vi "Move to point.vi"(11 "Point":T1) -> ()   [LabVIEW 2011]
uses:
  point.ctl
  <vilib>/addons/control/pid/pid.llb/PID (DBL).vi
  <vilib>/addons/control/pid/NI_PID_pid.lvlib
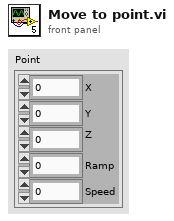
[diagram p1: front panel]
types:
  T1 = typedef "point.ctl" = cluster{"X":dbl, "Y":dbl, "Z":dbl, "Ramp":dbl, "Speed":dbl}
  T2 = typedef "WPI_EncoderDevRef.ctl" = cluster{"DevStatus":errorcluster, "EncoderIndex":T3, "CounterIndex":T4, "DistancePerCount":dbl, "Decoding Type":T5}
  T3 = typedef "FPGA_EncoderIdx.ctl" = enum8{"Enc 0", "Enc 1", "Enc 2", "Enc 3", "Invalid"}
  T4 = typedef "FPGA_CounterCtrSystemIndex.ctl" = enum8{"Ctr 0", "Ctr 1", "Ctr 2", "Ctr 3", "Ctr 4", "Ctr 5", "Ctr 6", "Ctr 7", "Invalid"}
  T5 = typedef "WPI_EncoderType.ctl" = enum16{"1x", "2x", "4x"}
  T6 = typedef "WPI_MotorControlDeviceRef.ctl" = cluster{"DeviceStatus":errorcluster, "Type":enum16{"PWM", "CAN"}, "PWM":cluster{"Digital Module":T7, "PWM Channel":T8, "DeadBand":T9}, "CAN":cluster{"Device Number":u8, "Control Mode":T10, "Semaphore":T11, "Max Vout":dbl}, "Invert":bool, "TransformRef":T12, "InvTransformRef":T12}
  T7 = typedef "FPGA_TypedefDigitalModule.ctl" = enum16{"Digital Module 1", "Digital Module 2"}
  T8 = typedef "FPGA_DIOPWMChannel.ctl" = enum8{"PWM 1", "PWM 2", "PWM 3", "PWM 4", "PWM 5", "PWM 6", "PWM 7", "PWM 8", "PWM 9", "PWM 10", "Invalid"}
  T9 = typedef "WPI_PWMDeadband.ctl" = cluster{"Name":string, "maxPositivePwm":i32, "minPositivePwm":i32, "centerPwm":i32, "maxNegativePwm":i32, "minNegativePwm":i32, "angularRange":u16}
  T10 = typedef "WPI_CANJaguar_ControlMode.ctl" = enum8{"Percent VBus", "Current", "Speed", "Position", "Voltage"}
  T11 = typedef "Semaphore RefNum" = refnum<k1>
  T12 = typedef "WPI_PWMTransform_ConPane.ctl" = refnum<vi>
  T13 = cluster{"proportional gain (Kc)":dbl, "integral time (Ti, min)":dbl, "derivative time (Td, min)":dbl}
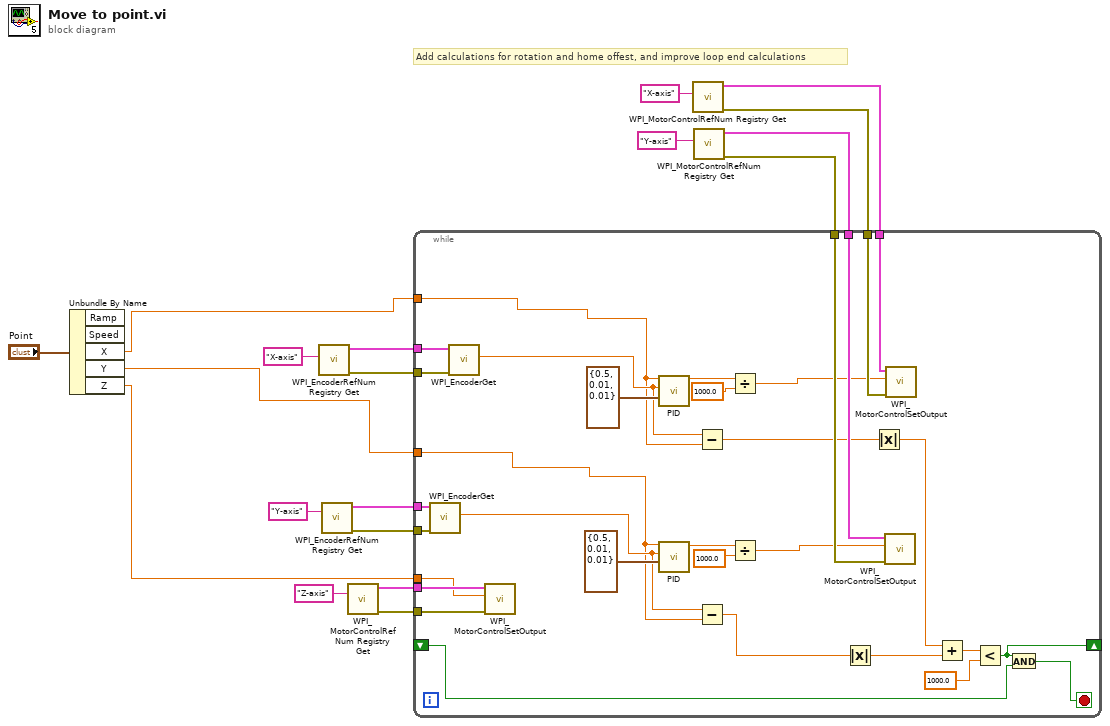
[diagram p0: block diagram]
diagram:
  # "Add calculations for rotation and home offest, and improve loop end calculations"
  n1 = Unbundle By Name("Point") -> ("X"=w1:dbl, "Y"=w2:dbl, "Z"=w3:dbl)  [unwired: 2 out]
  n2 = call <vilib>:"WPI_EncoderRefNum Registry Get.vi"("refnum name"="X-axis") -> ("error out"=w16:errorcluster, "EncoderDevRef"=w15:T2)  [unwired: 9 in]
  n3 = call <vilib>:"WPI_EncoderRefNum Registry Get.vi"("refnum name"="Y-axis") -> ("error out"=w13:errorcluster, "EncoderDevRef"=w14:T2)  [unwired: 9 in]
  n4 = call <vilib>:"WPI_MotorControlRefNum Registry Get.vi"("refnum name"="Z-axis") -> ("error out"=w5:errorcluster, "MotorControlDevRef"=w6:T6)  [unwired: 9 in]
  n5 = call <vilib>:"WPI_MotorControlRefNum Registry Get.vi"("refnum name"="X-axis") -> ("error out"=w10:errorcluster, "MotorControlDevRef"=w11:T6)  [unwired: 9 in]
  n6 = call <vilib>:"WPI_MotorControlRefNum Registry Get.vi"("refnum name"="Y-axis") -> ("error out"=w7:errorcluster, "MotorControlDevRef"=w8:T6)  [unwired: 9 in]
  n7 = while {
    tunnel: w1 -> [w22]
    tunnel: w16 -> [w49]
    tunnel: w15 -> [w48]
    tunnel: w2 -> [w23]
    tunnel: w14 -> [w45]
    tunnel: w13 -> [w44]
    shift-right: [w38] -> _
    shift-left: _ -> [w37]
    tunnel: w11 -> [w36]
    tunnel: w10 -> [w25]
    tunnel: w8 -> [w35]
    tunnel: w7 -> [w34]
    tunnel: w6 -> [w33]
    tunnel: w5 -> [w32]
    tunnel: w3 -> [w24]
    stop <- w26 stop-if-true
    n8 = call <vilib>:"WPI_EncoderGet.vi"("error in (no error)"=w44, "EncoderDevRef"=w45) -> ("Distance"=w27:dbl)  [unwired: 4 in, 5 out]
    n9 = call <vilib>:"WPI_EncoderGet.vi"("error in (no error)"=w49, "EncoderDevRef"=w48) -> ("Distance"=w31:dbl)  [unwired: 4 in, 5 out]
    n10 = call <vilib>:"WPI_MotorControlSetOutput.vi"("error in (no error)"=w32, "Output"=w24, "MotorControlDevRef"=w33) -> ()  [unwired: 7 in, 2 out]
    n11 = call-poly <vilib>:"PID.vi"("PID gains"=T13 {"proportional gain (Kc)"=0.5, "integral time (Ti, min)"=0.01, "derivative time (Td, min)"=0.01}, "process variable"=w31, "setpoint"=w22) -> ("output"=w42:dbl)  [unwired: 7 in, 1 out]
    n12 = call-poly <vilib>:"PID.vi"("PID gains"=T13 {"proportional gain (Kc)"=0.5, "integral time (Ti, min)"=0.01, "derivative time (Td, min)"=0.01}, "process variable"=w27, "setpoint"=w23) -> ("output"=w43:dbl)  [unwired: 7 in, 1 out]
    n13 = Subtract(x=w31, y=w22) -> (x-y=w29:dbl)
    n14 = Subtract(x=w27, y=w23) -> (x-y=w41:dbl)
    n15 = Divide(x=w42, y=1000.0) -> (x/y=w21:dbl)
    n16 = Divide(x=w43, y=1000.0) -> (x/y=w20:dbl)
    n17 = Absolute Value(x=w41) -> (abs(x)=w30:dbl)
    n18 = Absolute Value(x=w29) -> (abs(x)=w28:dbl)
    n19 = call <vilib>:"WPI_MotorControlSetOutput.vi"("error in (no error)"=w34, "Output"=w20, "MotorControlDevRef"=w35) -> ()  [unwired: 7 in, 2 out]
    n20 = call <vilib>:"WPI_MotorControlSetOutput.vi"("error in (no error)"=w25, "Output"=w21, "MotorControlDevRef"=w36) -> ()  [unwired: 7 in, 2 out]
    n21 = Add(x=w28, y=w30) -> (x+y=w40:dbl)
    n22 = Less?(x=w40, y=1000.0) -> (x < y?=w38:bool)
    n23 = And(x=w38, y=w37) -> (x .and. y?=w26:bool)
  }
